vi "VFP Network Set Buffering Attributes.vi"(9 "TypeDesc":T1, 10 "Ctl Ref Cluster":T3, 11 "attributes":T2) -> (3 "attributes out":T2)   [LabVIEW 2016]
uses:
  <resource>/dialog/variable/FeaturePacks/Network/VFP Network ControlRef.ctl
  <resource>/dialog/variable/SCT Attributes.ctl
  <vilib>/variable/Type Descriptor.ctl
  <vilib>/Utility/VariantDataType/Type.ctl
  <resource>/dialog/variable/FeaturePacks/Utility/VFP Util Fetch Bool Control.vi
  <vilib>/variable/NI_Variable.lvlib
  <vilib>/Utility/VariantDataType/VariantType.lvlib
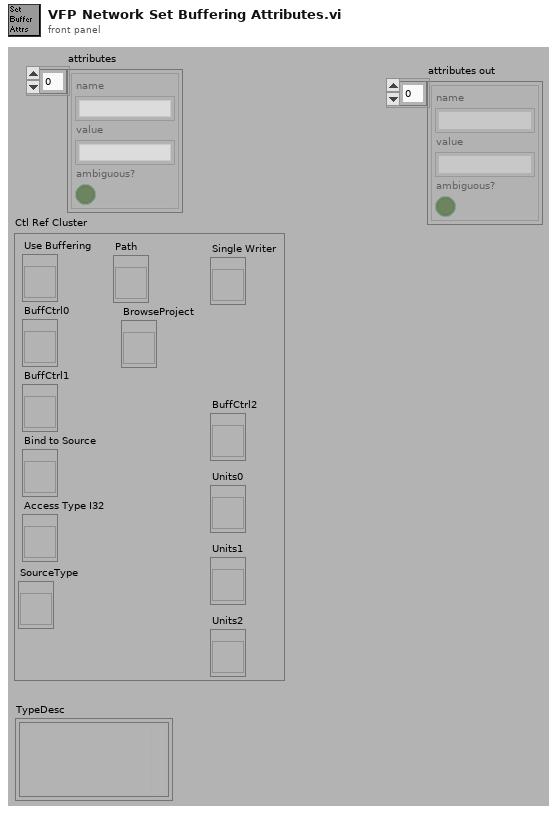
[diagram p1: front panel]
types:
  T1 = typedef "NI_Variable.lvlib/Type Descriptor.ctl" = cluster{"Variant":variant}
  T2 = typedef "SCT Attributes.ctl" = cluster{"name":string, "value":string, "ambiguous?":bool}[]
  T3 = typedef "VFP Network ControlRef.ctl" = cluster{"Use Buffering":refnum<vi>, "BuffCtrl0":refnum<vi>, "BuffCtrl1":refnum<vi>, "Bind to Source":refnum<vi>, "Access Type I32":refnum<vi>, "Path":refnum<vi>, "BrowseProject":refnum<vi>, "Single Writer":refnum<vi>, "BuffCtrl2":refnum<vi>, "Units0":refnum<vi>, "Units1":refnum<vi>, "Units2":refnum<vi>, "SourceType":refnum<vi>}
  T4 = typedef "VariantType.lvlib/Type.ctl" = enum8{"Invalid Type", "Void", "I8", "I16", "I32", "I64", "U8", "U16", "U32", "U64", "Single Float", "Double Float", "Extended Float", "Single Complex", "Double Complex", "Extended Complex", "Enum U8", "Enum U16", "Enum U32", "Enum U64", "Single Float With Unit", "Double Float With Unit", "Extended Float With Unit", "Single Complex with Unit", "Double Complex with Unit", "Extended Complex with Unit", "Boolean", "String", "Path", "Picture", "Tag", "Array", "Cluster", "Variant", "LV Variant", "Waveform", "Timestamp", "Digital Waveform", "Digital Data", "ExpressData", "Refnum", "External Data", "VI", "Poly VI", "LabVIEW Class Instance", "Fixed Point"}
  T5 = typedef "VFP Network Control Info.ctl" = cluster{"Label":string, "Unit":string, "Constant Value":cluster{"Constant Value":u32, "Constant?":bool}}
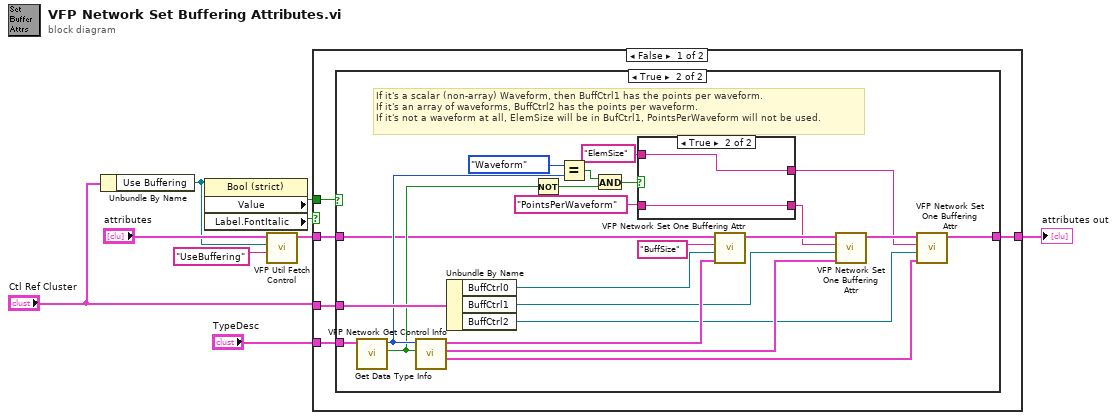
[diagram p0: block diagram]
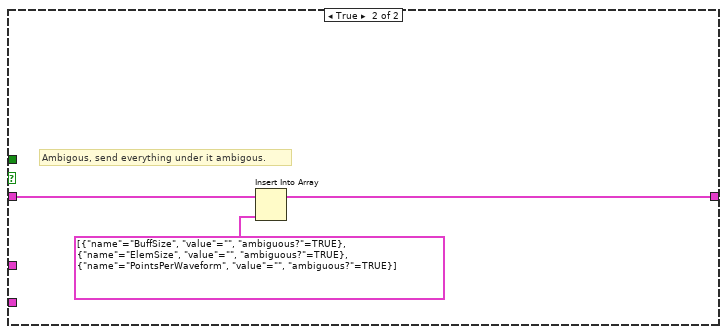
[diagram p4: hidden frame]
diagram:
  n1 = Unbundle By Name("Ctl Ref Cluster") -> ("Use Buffering"=w3:refnum<vi>)
  n2 = property class="Bool (strict)"(reference=w3) -> ("Value"=w8:bool, "Label.FontItalic"=w4:bool)  [unwired: 1 in, 2 out]
  n3 = call-poly <resource>:"VFP Util Fetch Control.vi"("attribute name"="UseBuffering", "control"=w3, "attributes"="attributes") -> ("attributes out"=w5:T2)  [unwired: 7 in, 1 out]
  n4 = case shown="False" w4 {
    tunnel: "TypeDesc" -> [w14 _]
    tunnel: w5 -> [w10 w45]
    tunnel: [w13 w43] -> w6
    tunnel: w8 -> [w12 _]
    tunnel: "Ctl Ref Cluster" -> [w11 _]
    frame False {
      n5 = case shown="True" w12 {
        tunnel: w14 -> [_ w38]
        tunnel: [w15 w16] -> w13
        tunnel: w11 -> [_ w37]
        tunnel: w10 -> [w15 w31]
        frame False {
          # "No Buffering, do not even write the rest of attributes."
        }
        frame True {
          # "If it's a scalar (non-array) Waveform, then BuffCtrl1 has the points per waveform.\nIf it's an array of waveforms, BuffCtrl2 has the points per waveform.\nIf it's not a waveform at all, ElemSize will be in BufCtrl1, PointsPerWaveform will not be used."
          n6 = call <vilib>:"Get Data Type Info.vi"("TypeDesc"=w38) -> ("Is Array?"=w34:bool, "Fundamental Type"=w36:T4)  [unwired: 9 in]
          n7 = call <resource>:"VFP Network Get Control Info.vi"("Is Array?"=w34, "Fundamental Type"=w36) -> ("BuffCtrl2 Info"=w25:T5, "BuffCtrl1 Info"=w27:T5, "BuffCtrl0 Info"=w29:T5)  [unwired: 7 in]
          n8 = Unbundle By Name(w37) -> ("BuffCtrl0"=w30:refnum<vi>, "BuffCtrl1"=w24:refnum<vi>, "BuffCtrl2"=w23:refnum<vi>)
          n9 = Not(x=w34) -> (.not. x?=w32:bool)
          n10 = Equal?(x=Type."Waveform" ("y"), y=w36) -> (x = y?=w33:bool)
          n11 = And(x=w33, y=w32) -> (x .and. y?=w21:bool)
          n12 = case shown="True" w21 {
            tunnel: "PointsPerWaveform" ("attribute name") -> [w39 w41]
            tunnel: [w39 w42] -> w17
            tunnel: "ElemSize" ("attribute name") -> [w40 w42]
            tunnel: [w40 w41] -> w18
            frame False {
            }
            frame True {
            }
          }
          n13 = call <resource>:"VFP Network Set One Buffering Attr.vi"("Ctrl Info"=w29, "Ctrl Ref"=w30, "attribute name"="BuffSize", "attributes in"=w31) -> ("attributes out"=w28:T2)  [unwired: 7 in]
          n14 = call <resource>:"VFP Network Set One Buffering Attr.vi"("Ctrl Info"=w27, "Ctrl Ref"=w24, "attribute name"=w18, "attributes in"=w28) -> ("attributes out"=w26:T2)  [unwired: 7 in]
          n15 = call <resource>:"VFP Network Set One Buffering Attr.vi"("Ctrl Info"=w25, "Ctrl Ref"=w23, "attribute name"=w17, "attributes in"=w26) -> ("attributes out"=w16:T2)  [unwired: 7 in]
        }
      }
    }
    frame True {
      # "Ambigous, send everything under it ambigous."
      n16 = Insert Into Array(array=w45, new element=T2 [{"name"="BuffSize", "value"="", "ambiguous?"=TRUE}, {"name"="ElemSize", "value"="", "ambiguous?"=TRUE}, {"name"="PointsPerWaveform", "value"="", "ambiguous?"=TRUE}] ("attributes")) -> (w43:T2)  [unwired: 1 in]
    }
  }
  "attributes out" <- w6
